vi "pixel to wavelength using cal array.vi"(10 "Cal array":dbl[](array[numeric]), 11 "# pix":i32) -> (3 "Wavelength Array":dbl[](array[numeric]))   [LabVIEW 2013]
panel:
  out "sum 3":dbl
  out "sum 2":dbl
  out "sum":dbl
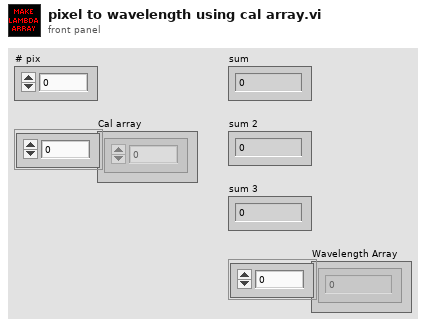
[diagram p1: front panel]
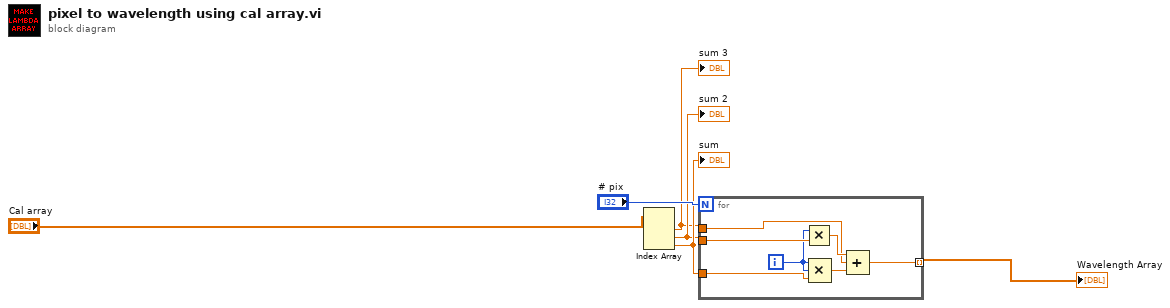
[diagram p0: block diagram]
diagram:
  n1 = Index Array(array="Cal array") -> (element #1=w1:dbl, element #2=w2:dbl, element #3=w3:dbl)  [unwired: 3 in]
  "sum" <- w3
  "sum 2" <- w2
  "sum 3" <- w1
  n2 = for {
    N: "# pix" -> [_]
    tunnel: [w7] -> w5 mode=indexing
    tunnel: w2 -> [w12]
    tunnel: w1 -> [w11]
    tunnel: w3 -> [w9]
    i -> [w10]
    n3 = Multiply(x=w10, y=w12) -> (x*y=w13:dbl)
    n4 = Compound Arithmetic op=MULTIPLY(w10, w10, w9) -> (w8:dbl)
    n5 = Compound Arithmetic op=ADD(w13, w11, w8) -> (w7:dbl)
  }
  "Wavelength Array" <- w5
